vi "del_fs_to_del_mm.vi"(2 "Delays / fs":dbl[](array[numeric])=[-500.0, -250.0, -100.0, -50.0, -25.0, 0.0, 25.0, 50.0, 100.0, 250.0, 1000.0, 3000.0, 5000.0], 3 "t0 / mm":dbl) -> (1 "Delays / mm":dbl[](array[numeric]))   [LabVIEW 2019]
doc: "Given a list of delays in femtoseconds and to in mm, converts delays into mm"
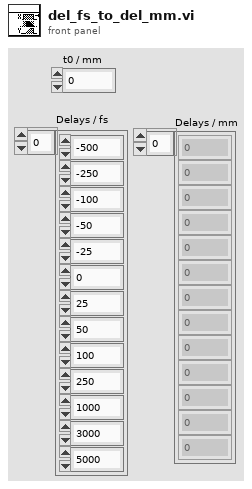
[diagram p1: front panel]
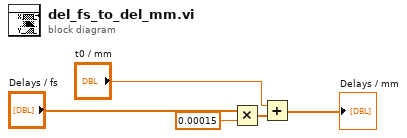
[diagram p0: block diagram]
diagram:
  n1 = Multiply(x="Delays / fs", y=0.00015 ("Numeric")) -> (x*y=w3:dbl[])
  n2 = Add(x="t0 / mm", y=w3) -> (x+y=→"Delays / mm":dbl[])
